vi "Verify Parameterized.vi"(5 "Label":string, 7 "Options":refnum<class "Options.lvclass">, 8 "error in":errorcluster, 9 "Set of ctl label -> value var":set{map{string, variant}}(c389), 10 "VI in":refnum<vi>, 11 "LUnit Test Case In":refnum<class "Test Case.lvclass">) -> (0 "error out":errorcluster, 3 "LUnit Test Case Out":refnum<class "Test Case.lvclass">)   [LabVIEW 2020, in "LUnit.Extension.lvlib"]
doc: "You pass in a reference to the function you want to test. You also pass in a set of maps. Each map maps each control label to a variant value (You must use the \"to Variant\" primitive or you'll get a broken run arrow due to the type mismatch). The control must be connected to the connector pane. Ideally you would have the same number of elements in your map as controls connected to the connector pane. If you don't specify a value for a control, it just stays whatever the default is set at. The underlying code will cycle through the set and for each map, will set the control values appropriately and then run the vi and capture any indicators connected to the connector pane. The control and corresponding indicator values are all stored in the approved file."
uses:
  LUnit.Extension.lvlib
  <vilib>/Astemes/LUnit/Test Case.lvclass
  Approval Tests/Options/Options.lvclass
  Approval Tests/Options/Options.lvclass/Options.ctl
  Approval Tests/Naming Data/Naming Data.lvclass/Naming Data.ctl
  <vilib>/Astemes/LUnit/Test Case.lvclass/Test Case.ctl
  Approval Tests/Naming Data/Read Test VI Name.vi
  Approval Tests/Naming Data/Write Test VI Name.vi
  <vilib>/Astemes/LUnit/Core/LUnit Test Case/Private/Append Fail Result.vi
  <vilib>/Astemes/LUnit/Core/LUnit Test Case/Private/Append Pass Result.vi
  <vilib>/Astemes/LUnit/Core/LUnit Test Case/Private/Run In UI.vi
  <vilib>/Utility/error.llb/Clear Errors.vi
  Approval Tests/Approval Tests.lvlib
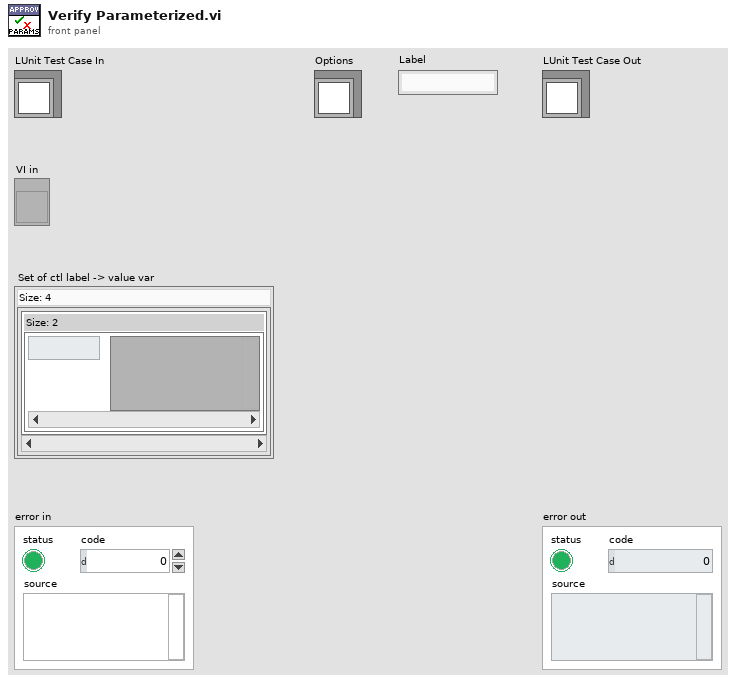
[diagram p1: front panel]
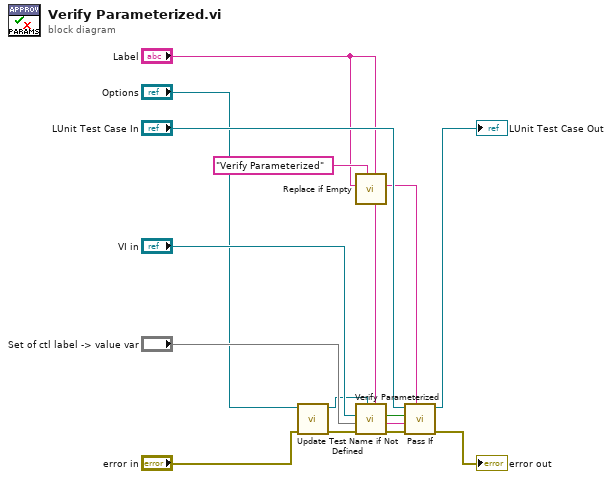
[diagram p0: block diagram]
diagram:
  n1 = call "Update Test Name if Not Defined.vi"("error in"="error in", "Options in"="Options") -> ("error out"=w12:errorcluster, "Options out"=w4:refnum<class "Options.lvclass">)  [unwired: 8 in]
  n2 = call "Replace if Empty.vi"("if empty"="Verify Parameterized", "Text in"="Label") -> ("Text out"=w1:string)  [unwired: 9 in]
  n3 = call "Verify Parameterized.vi"("Label"="Label", "Approval Tests.lvlib:Options.lvclass"=w4, "error in"=w12, "Set of ctl label -> value var"="Set of ctl label -> value var", "VI in"="VI in") -> ("error out"=w13:errorcluster, "Failure Message"=w8:string, "Passed?"=w9:bool)  [unwired: 4 in]
  n4 = call <vilib>:"Pass If.vi"("Description"=w1, "error in (no error)"=w13, "Message"=w8, "Pass?"=w9, "LUnit Test Case In"="LUnit Test Case In") -> ("error out"=→"error out":errorcluster, "LUnit Test Case Out"=→"LUnit Test Case Out":refnum<class "Test Case.lvclass">)  [unwired: 5 in]
